vi "Func-엑셀 데이터를 그래프로 출력.vi"() -> ()   [LabVIEW 2015] (continued)
-18.31\t-7.631\n-18.3\t-18.31\t-7.633\n-18.3\t-18.31\t-7.634\n-18.3\t-18.31\t-7.636\n-18.3\t-18.31\t-7.633\n-18.3\t-18.31\t-7.632\n-18.3\t-18.31\t-7.636\n-18.3\t-18.31\t-7.635\n-18.3\t-18.31\t-7.636\n-18.3\t-18.31\t-7.638\n-18.3\t-18.31\t-7.643\n-18.3\t-18.31\t-7.647\n-18.3\t-18.31\t-7.651\n-18.3\t-18.31\t-7.656\n-18.3\t-18.31\t-7.657\n-18.3\t-18.31\t-7.659\n-18.3\t-18.31\t-7.66\n-18.3\t-18.31\t-7.66\n-18.3\t-18.31\t-7.657\n-18.3\t-18.31\t-7.656\n-18.3\t-18.31\t-7.662\n-18.3\t-18.31\t-7.664\n-18.3\t-18.31\t-7.667\n-18.3\t-18.31\t-7.672\n-18.3\t-18.31\t-7.676\n-18.3\t-18.31\t-7.674\n-18.3\t-18.31\t-7.676\n-18.3\t-18.31\t-7.677\n-18.3\t-18.31\t-7.675\n-18.3\t-18.31\t-7.674\n-18.3\t-18.31\t-7.675\n-18.3\t-18.31\t-7.681\n-18.3\t-18.31\t-7.683\n-18.3\t-18.31\t-7.687\n-18.3\t-18.31\t-7.689\n-18.3\t-18.31\t-7.693\n-18.3\t-18.31\t-7.695\n-18.3\t-18.31\t-7.696\n-18.3\t-18.31\t-7.696\n-18.3\t-18.31\t-7.693\n-18.3\t-18.31\t-7.695\n-18.3\t-18.31\t-7.694\n-18.3\t-18.31\t-7.695\n-18.3\t-18.31\t-7.696\n-18.3\t-18.31\t-7.699\n-18.3\t-18.31\t-7.702\n-18.3\t-18.31\t-7.704\n-18.3\t-18.31\t-7.707\n-18.3\t-18.31\t-7.707\n-18.3\t-18.31\t-7.709\n-18.3\t-18.31\t-7.711\n-18.3\t-18.31\t-7.711\n-18.3\t-18.31\t-7.714\n-18.3\t-18.31\t-7.716\n-18.3\t-18.31\t-7.72\n-18.3\t-18.31\t-7.723\n-18.3\t-18.31\t-7.727\n-18.3\t-18.31\t-7.728\n-18.3\t-18.31\t-7.729\n-18.3\t-18.31\t-7.732\n-18.3\t-18.31\t-7.731\n-18.3\t-18.31\t-7.73\n-18.3\t-18.31\t-7.729\n-18.3\t-18.31\t-7.729\n-18.3\t-18.31\t-7.73\n-18.3\t-18.31\t-7.731\n-18.3\t-18.31\t-7.73\n-18.3\t-18.31\t-7.732\n-18.3\t-18.31\t-7.734\n-18.3\t-18.31\t-7.74\n-18.3\t-18.31\t-7.743\n-18.3\t-18.31\t-7.744\n-18.3\t-18.31\t-7.747\n-18.3\t-18.31\t-7.746\n-18.3\t-18.31\t-7.745\n-18.3\t-18.31\t-7.743\n-18.3\t-18.31\t-7.745\n-18.3\t-18.31\t-7.747\n-18.3\t-18.31\t-7.746\n-18.3\t-18.31\t-7.752\n-18.3\t-18.31\t-7.754\n-18.3\t-18.31\t-7.759\n-18.3\t-18.31\t-7.761\n-18.3\t-18.31\t-7.765\n-18.3\t-18.31\t-7.765\n-18.3\t-18.31\t-7.766\n-18.3\t-18.31\t-7.766\n-18.3\t-18.31\t-7.764\n-18.3\t-18.31\t-7.764\n-18.3\t-18.31\t-7.76\n-18.3\t-18.31\t-7.767\n-18.3\t-18.31\t-7.767\n-18.3\t-18.31\t-7.768\n-18.3\t-18.31\t-7.77\n-18.3\t-18.31\t-7.772\n-18.3\t-18.31\t-7.776\n-18.3\t-18.31\t-7.777\n-18.3\t-18.31\t-7.777\n-18.3\t-18.31\t-7.779\n-18.3\t-18.31\t-7.781\n-18.3\t-18.31\t-7.782\n-18.3\t-18.31\t-7.785\n-18.3\t-18.31\t-7.787\n-18.3\t-18.31\t-7.792\n-18.3\t-18.31\t-7.796\n-18.3\t-18.31\t-7.798\n-18.3\t-18.31\t-7.801\n-18.3\t-18.31\t-7.799\n-18.3\t-18.31\t-7.797\n-18.3\t-18.31\t-7.796\n-18.3\t-18.31\t-7.794\n-18.3\t-18.31\t-7.796\n-18.3\t-18.31\t-7.796\n-18.3\t-18.31\t-7.8\n-18.3\t-18.31\t-7.805\n-18.3\t-18.31\t-7.808\n-18.3\t-18.31\t-7.809\n-18.3\t-18.31\t-7.809\n-18.3\t-18.31\t-7.808\n-18.3\t-18.31\t-7.808\n-18.3\t-18.31\t-7.809\n-18.3\t-18.31\t-7.812\n-18.3\t-18.31\t-7.813\n-18.3\t-18.31\t-7.817\n-18.3\t-18.31\t-7.82\n-18.3\t-18.31\t-7.821\n-18.3\t-18.31\t-7.825\n-18.3\t-18.31\t-7.823\n-18.3\t-18.31\t-7.824\n-18.3\t-18.31\t-7.827\n-18.3\t-18.31\t-7.827\n-18.3\t-18.31\t-7.828\n-18.3\t-18.31\t-7.828\n-18.3\t-18.31\t-7.829\n-18.3\t-18.31\t-7.834\n-18.3\t-18.31\t-7.836\n-18.3\t-18.31\t-7.836\n-18.3\t-18.31\t-7.838\n-18.3\t-18.31\t-7.838\n-18.3\t-18.31\t-7.839\n-18.3\t-18.31\t-7.838\n-18.3\t-18.31\t-7.839\n-18.3\t-18.31\t-7.84\n-18.3\t-18.31\t-7.841\n-18.3\t-18.31\t-7.847\n-18.3\t-18.31\t-7.852\n-18.3\t-18.31\t-7.852\n-18.3\t-18.31\t-7.852\n-18.3\t-18.31\t-7.858\n-18.3\t-18.31\t-7.863\n-18.3\t-18.31\t-7.859\n-18.3\t-18.31\t-7.857\n-18.3\t-18.31\t-7.858\n-18.3\t-18.31\t-7.866\n-18.3\t-18.31\t-7.859\n-18.3\t-18.31\t-7.858\n-18.3\t-18.31\t-7.86\n-18.3\t-18.31\t-7.863\n-18.3\t-18.31\t-7.864\n-18.3\t-18.31\t-7.863\n-18.3\t-18.31\t-7.87\n-18.3\t-18.31\t-7.87\n-18.3\t-18.31\t-7.875\n-18.3\t-18.31\t-7.876\n-18.3\t-18.31\t-7.877\n-18.3\t-18.31\t-7.877\n-18.3\t-18.31\t-7.878\n-18.3\t-18.31\t-7.877\n-18.3\t-18.31\t-7.875\n-18.3\t-18.31\t-7.878\n-18.3\t-18.31\t-7.88\n-18.3\t-18.31\t-7.883\n-18.3\t-18.31\t-7.886\n-18.3\t-18.31\t-7.891\n-18.3\t-18.31\t-7.889\n-18.3\t-18.31\t-7.887\n-18.3\t-18.31\t-7.889\n-18.3\t-18.31\t-7.888\n-18.3\t-18.31\t-7.888\n-18.3\t-18.31\t-7.888\n-18.3\t-18.31\t-7.894\n-18.3\t-18.31\t-7.893\n-18.3\t-18.31\t-7.895\n-18.3\t-18.31\t-7.896\n-18.3\t-18.31\t-7.897\n-18.3\t-18.31\t-7.898\n-18.3\t-18.31\t-7.899\n-18.3\t-18.31\t-7.904\n-18.3\t-18.31\t-7.904\n-18.3\t-18.31\t-7.904\n-18.3\t-18.31\t-7.903\n-18.3\t-18.31\t-7.905\n-18.3\t-18.31\t-7.905\n-18.3\t-18.31\t-7.904\n-18.3\t-18.31\t-7.905\n-18.3\t-18.31\t-7.902\n-18.3\t-18.31\t-7.904\n-18.3\t-18.31\t-7.903\n-18.3\t-18.31\t-7.905\n-18.3\t-18.31\t-7.907\n-18.3\t-18.31\t-7.909\n-18.3\t-18.31\t-7.914\n-18.3\t-18.31\t-7.914\n-18.3\t-18.31\t-7.922\n-18.3\t-18.31\t-7.925\n-18.3\t-18.31\t-7.925\n-18.3\t-18.31\t-7.929\n-18.3\t-18.31\t-7.925\n-18.3\t-18.31\t-7.926\n-18.3\t-18.31\t-7.925\n-18.3\t-18.31\t-7.925\n-18.3\t-18.31\t-7.926\n-18.3\t-18.31\t-7.926\n-18.3\t-18.31\t-7.933\n-18.3\t-18.31\t-7.938\n-18.3\t-18.31\t-7.938\n-18.3\t-18.31\t-7.942\n-18.3\t-18.31\t-7.946\n-18.3\t-18.31\t-7.947\n-18.3\t-18.31\t-7.944\n-18.3\t-18.31\t-7.946\n-18.3\t-18.31\t-7.946\n-18.3\t-18.31\t-7.943\n-18.3\t-18.31\t-7.942\n-18.3\t-18.31\t-7.945\n-18.3\t-18.31\t-7.95\n-18.3\t-18.31\t-7.948\n-18.3\t-18.31\t-7.95\n-18.3\t-18.31\t-7.951\n-18.3\t-18.31\t-7.952\n-18.3\t-18.31\t-7.951\n-18.3\t-18.31\t-7.951\n-18.3\t-18.31\t-7.954\n-18.3\t-18.31\t-7.954\n-18.3\t-18.31\t-7.957\n-18.3\t-18.31\t-7.958\n-18.3\t-18.31\t-7.96\n-18.3\t-18.31\t-7.959\n-18.3\t-18.31\t-7.957\n-18.3\t-18.31\t-7.962\n-18.3\t-18.31\t-7.96\n-18.3\t-18.31\t-7.961\n-18.3\t-18.31\t-7.964\n-18.3\t-18.31\t-7.968\n-18.3\t-18.31\t-7.972\n-18.3\t-18.31\t-7.971\n-18.3\t-18.31\t-7.974\n-18.3\t-18.31\t-7.974\n-18.3\t-18.31\t-7.973\n-18.3\t-18.31\t-7.974\n-18.3\t-18.31\t-7.975\n-18.3\t-18.31\t-7.978\n-18.3\t-18.31\t-7.979\n-18.3\t-18.31\t-7.978\n-18.3\t-18.31\t-7.981\n-18.3\t-18.31\t-7.981\n-18.3\t-18.31\t-7.98\n-18.3\t-18.31\t-7.982\n-18.3\t-18.31\t-7.984\n-18.3\t-18.31\t-7.987\n-18.3\t-18.31\t-7.989\n-18.3\t-18.31\t-7.992\n-18.3\t-18.31\t-7.99\n-18.3\t-18.31\t-7.989\n-18.3\t-18.31\t-7.988\n-18.3\t-18.31\t-7.991\n-18.3\t-18.31\t-7.988\n-18.3\t-18.31\t-7.988\n-18.3\t-18.31\t-7.995\n-18.3\t-18.31\t-8\n-18.3\t-18.31\t-7.999\n-18.3\t-18.31\t-7.998\n-18.3\t-18.31\t-8.001\n-18.3\t-18.31\t-8.003\n-18.3\t-18.31\t-8.003\n-18.3\t-18.31\t-8.001\n-18.3\t-18.31\t-8.005\n-18.3\t-18.31\t-8.007\n-18.3\t-18.31\t-8.007\n-18.3\t-18.31\t-8.009\n-18.3\t-18.31\t-8.009\n-18.3\t-18.31\t-8.011\n-18.3\t-18.31\t-8.01\n-18.3\t-18.31\t-8.01\n-18.3\t-18.31\t-8.013\n-18.3\t-18.31\t-8.01\n-18.3\t-18.31\t-8.011\n-18.3\t-18.31\t-8.014\n-18.3\t-18.31\t-8.013\n-18.3\t-18.31\t-8.016\n-18.3\t-18.31\t-8.017\n-18.3\t-18.31\t-8.018\n-18.3\t-18.31\t-8.021\n-18.3\t-18.31\t-8.023\n-18.3\t-18.31\t-8.025\n-18.3\t-18.31\t-8.026\n-18.3\t-18.31\t-8.029\n-18.3\t-18.31\t-8.03\n-18.3\t-18.31\t-8.028\n-18.3\t-18.31\t-8.025\n-18.3\t-18.31\t-8.028\n-18.3\t-18.31\t-8.032\n-18.3\t-18.31\t-8.03\n-18.3\t-18.31\t-8.03\n-18.3\t-18.31\t-8.033\n-18.3\t-18.31\t-8.034\n-18.3\t-18.31\t-8.034\n-18.3\t-18.31\t-8.03\n-18.3\t-18.31\t-8.032\n-18.3\t-18.31\t-8.036\n-18.3\t-18.31\t-8.04\n-18.3\t-18.31\t-8.041\n-18.3\t-18.31\t-8.043\n-18.3\t-18.31\t-8.046\n-18.3\t-18.31\t-8.043\n-18.3\t-18.31\t-8.042\n-18.3\t-18.31\t-8.043\n-18.3\t-18.31\t-8.046\n-18.3\t-18.31\t-8.048\n-18.3\t-18.31\t-8.049\n-18.3\t-18.31\t-8.055\n-18.3\t-18.31\t-8.056\n-18.3\t-18.31\t-8.059\n-18.3\t-18.31\t-8.061\n-18.3\t-18.31\t-8.06\n-18.3\t-18.31\t-8.062\n-18.3\t-18.31\t-8.06\n-18.3\t-18.31\t-8.061\n-18.3\t-18.31\t-8.061\n-18.3\t-18.31\t-8.064\n-18.3\t-18.31\t-8.066\n-18.3\t-18.31\t-8.068\n-18.3\t-18.31\t-8.068\n-18.3\t-18.31\t-8.068\n-18.3\t-18.31\t-8.067\n-18.3\t-18.31\t-8.065\n-18.3\t-18.31\t-8.064\n-18.3\t-18.31\t-8.068\n-18.3\t-18.31\t-8.066\n-18.3\t-18.31\t-8.066\n-18.3\t-18.31\t-8.069\n-18.3\t-18.31\t-8.07\n-18.3\t-18.31\t-8.071\n-18.3\t-18.31\t-8.068\n-18.3\t-18.31\t-8.074\n-18.3\t-18.31\t-8.079\n-18.3\t-18.31\t-8.08\n-18.3\t-18.31\t-8.081\n-18.3\t-18.31\t-8.082\n-18.3\t-18.31\t-8.084\n-18.3\t-18.31\t-8.082\n-18.3\t-18.31\t-8.08\n-18.3\t-18.31\t-8.08\n-18.3\t-18.31\t-8.078\n-18.3\t-18.31\t-8.082\n-18.3\t-18.31\t-8.086\n-18.3\t-18.31\t-8.089\n-18.3\t-18.31\t-8.093\n-18.3\t-18.31\t-8.095\n-18.3\t-18.31\t-8.098\n-18.3\t-18.31\t-8.096\n-18.3\t-18.31\t-8.097\n-18.3\t-18.31\t-8.095\n-18.3\t-18.31\t-8.097\n-18.3\t-18.31\t-8.099\n-18.3\t-18.31\t-8.098\n-18.3\t-18.31\t-8.1\n-18.3\t-18.31\t-8.1\n-18.3\t-18.31\t-8.1\n-18.3\t-18.31\t-8.097\n-18.3\t-18.31\t-8.094\n-18.3\t-18.31\t-8.096\n-18.3\t-18.31\t-8.098\n-18.3\t-18.31\t-8.097\n-18.3\t-18.31\t-8.101\n-18.3\t-18.31\t-8.105\n-18.3\t-18.31\t-8.108\n-18.3\t-18.31\t-8.11\n-18.3\t-18.31\t-8.111\n-18.3\t-18.31\t-8.113\n-18.3\t-18.31\t-8.116\n-18.3\t-18.31\t-8.117\n-18.3\t-18.31\t-8.117\n-18.3\t-18.31\t-8.117\n-18.3\t-18.31\t-8.116\n-18.3\t-18.31\t-8.118\n-18.3\t-18.31\t-8.12\n-18.3\t-18.31\t-8.125\n-18.3\t-18.31\t-8.125\n-18.3\t-18.31\t-8.127\n-18.3\t-18.31\t-8.132\n-18.3\t-18.31\t-8.131\n-18.3\t-18.31\t-8.13\n-18.3\t-18.31\t-8.128\n-18.3\t-18.31\t-8.129\n-18.3\t-18.31\t-8.125\n-18.3\t-18.31\t-8.125\n-18.3\t-18.31\t-8.125\n-18.3\t-18.31\t-8.124\n-18.3\t-18.31\t-8.126\n-18.3\t-18.31\t-8.126\n-18.3\t-18.31\t-8.132\n-18.3\t-18.31\t-8.134\n-18.3\t-18.31\t-8.136\n-18.3\t-18.31\t-8.136\n-18.3\t-18.31\t-8.134\n-18.3\t-18.31\t-8.136\n-18.3\t-18.31\t-8.132\n-18.3\t-18.31\t-8.13\n-18.3\t-18.31\t-8.131\n-18.3\t-18.31\t-8.135\n-18.3\t-18.31\t-8.139\n-18.3\t-18.31\t-8.138\n-18.3\t-18.31\t-8.14\n-18.3\t-18.31\t-8.143\n-18.3\t-18.31\t-8.144\n-18.3\t-18.31\t-8.144\n-18.3\t-18.31\t-8.145\n-18.3\t-18.31\t-8.145\n-18.3\t-18.31\t-8.149\n-18.3\t-18.31\t-8.15\n-18.3\t-18.31\t-8.148\n-18.3\t-18.31\t-8.148\n-18.3\t-18.31\t-8.145\n-18.3\t-18.31\t-8.147\n-18.3\t-18.31\t-8.146\n-18.3\t-18.31\t-8.15\n-18.3\t-18.31\t-8.154\n-18.3\t-18.31\t-8.154\n-18.3\t-18.31\t-8.16\n-18.3\t-18.31\t-8.16\n-18.3\t-18.31\t-8.159\n-18.3\t-18.31\t-8.158\n-18.3\t-18.31\t-8.154\n-18.3\t-18.31\t-8.155\n-18.3\t-18.31\t-8.155\n-18.3\t-18.31\t-8.157\n-18.3\t-18.31\t-8.159\n-18.3\t-18.31\t-8.159\n-18.3\t-18.31\t-8.161\n-18.3\t-18.31\t-8.163\n-18.3\t-18.31\t-8.162\n-18.3\t-18.31\t-8.163\n-18.3\t-18.31\t-8.164\n-18.3\t-18.31\t-8.164\n-18.3\t-18.31\t-8.168\n-18.3\t-18.31\t-8.166\n-18.3\t-18.31\t-8.168\n-18.3\t-18.31\t-8.17\n-18.3\t-18.31\t-8.174\n-18.3\t-18.31\t-8.174\n-18.3\t-18.31\t-8.174\n-18.3\t-18.31\t-8.177\n-18.3\t-18.31\t-8.18\n-18.3\t-18.31\t-8.181\n-18.3\t-18.31\t-8.179\n-18.3\t-18.31\t-8.178\n-18.3\t-18.31\t-8.177\n-18.3\t-18.31\t-8.178\n-18.3\t-18.31\t-8.177\n-18.3\t-18.31\t-8.175\n-18.3\t-18.31\t-8.178\n-18.3\t-18.31\t-8.181\n-18.3\t-18.31\t-8.186\n-18.3\t-18.31\t-8.185\n-18.3\t-18.31\t-8.188\n-18.3\t-18.31\t-8.189\n-18.3\t-18.31\t-8.189\n-18.3\t-18.31\t-8.186\n-18.3\t-18.31\t-8.184\n-18.3\t-18.31\t-8.187\n-18.3\t-18.31\t-8.187\n-18.3\t-18.31\t-8.189\n-18.3\t-18.31\t-8.19\n-18.3\t-18.31\t-8.195\n-18.3\t-18.31\t-8.197\n-18.3\t-18.31\t-8.197\n-18.3\t-18.31\t-8.196\n-18.3\t-18.31\t-8.197\n-18.3\t-18.31\t-8.198\n-18.3\t-18.31\t-8.201\n-18.3\t-18.31\t-8.202\n-18.3\t-18.31\t-8.205\n-18.3\t-18.31\t-8.207\n-18.3\t-18.31\t-8.209\n-18.3\t-18.31\t-8.211\n-18.3\t-18.31\t-8.209\n-18.3\t-18.31\t-8.211\n-18.3\t-18.31\t-8.209\n-18.3\t-18.31\t-8.207\n-18.3\t-18.31\t-8.21\n-18.3\t-18.31\t-8.212\n-18.3\t-18.31\t-8.216\n-18.3\t-18.31\t-8.216\n-18.3\t-18.31\t-8.215\n-18.3\t-18.31\t-8.22\n-18.3\t-18.31\t-8.218\n-18.3\t-18.31\t-8.214\n-18.3\t-18.31\t-8.214\n-18.3\t-18.31\t-8.213\n-18.3\t-18.31\t-8.214\n-18.3\t-18.31\t-8.213\n-18.3\t-18.31\t-8.213\n-18.3\t-18.31\t-8.218\n-18.3\t-18.31\t-8.218\n-18.3\t-18.31\t-8.22\n-18.3\t-18.31\t-8.226\n-18.3\t-18.31\t-8.226\n-18.3\t-18.31\t-8.229\n-18.3\t-18.31\t-8.229\n-18.3\t-18.31\t-8.229\n-18.3\t-18.31\t-8.229\n-18.3\t-18.31\t-8.226\n-18.3\t-18.31\t-8.226\n-18.3\t-18.31\t-8.224\n-18.3\t-18.31\t-8.221\n-18.3\t-18.31\t-8.225\n-18.3\t-18.31\t-8.225\n-18.3\t-18.31\t-8.233\n-18.3\t-18.31\t-8.232\n-18.3\t-18.31\t-8.234\n-18.3\t-18.31\t-8.238\n-18.3\t-18.31\t-8.235\n-18.3\t-18.31\t-8.236\n-18.3\t-18.31\t-8.23\n-18.3\t-18.31\t-8.234\n-18.3\t-18.31\t-8.234\n-18.3\t-18.31\t-8.233\n-18.3\t-18.31\t-8.237\n-18.3\t-18.31\t-8.239\n-18.3\t-18.31\t-8.241\n-18.3\t-18.31\t-8.24\n-18.3\t-18.31\t-8.24\n-18.3\t-18.31\t-8.241\n-18.3\t-18.31\t-8.241\n-18.3\t-18.31\t-8.243\n-18.3\t-18.31\t-8.244\n-18.3\t-18.31\t-8.245\n-18.3\t-18.31\t-8.249\n-18.3\t-18.31\t-8.251\n-18.3\t-18.31\t-8.248\n-18.3\t-18.31\t-8.245\n-18.3\t-18.31\t-8.249\n-18.3\t-18.31\t-8.252\n-18.3\t-18.31\t-8.25\n-18.3\t-18.31\t-8.251\n-18.3\t-18.31\t-8.253\n-18.3\t-18.31\t-8.255\n-18.3\t-18.31\t-8.254\n-18.3\t-18.31\t-8.254\n-18.3\t-18.31\t-8.254\n-18.3\t-18.31\t-8.257\n-18.3\t-18.31\t-8.258\n-18.3\t-18.31\t-8.257\n-18.3\t-18.31\t-8.259\n-18.3\t-18.31\t-8.262\n-18.3\t-18.31\t-8.265\n-18.3\t-18.31\t-8.263\n-18.3\t-18.31\t-8.265\n-18.3\t-18.31\t-8.268\n-18.3\t-18.31\t-8.272\n-18.3\t-18.31\t-8.272\n-18.3\t-18.31\t-8.272\n-18.3\t-18.31\t-8.272\n-18.3\t-18.31\t-8.271\n-18.3\t-18.31\t-8.268\n-18.3\t-18.31\t-8.266\n-18.3\t-18.31\t-8.268\n-18.3\t-18.31\t-8.27\n-18.3\t-18.31\t-8.273\n-18.3\t-18.31\t-8.273\n-18.3\t-18.31\t-8.275\n-18.3\t-18.31\t-8.273\n-18.3\t-18.31\t-8.271\n-18.3\t-18.31\t-8.273\n-18.3\t-18.31\t-8.277\n-18.3\t-18.31\t-8.279\n-18.3\t-18.31\t-8.28\n-18.3\t-18.31\t-8.287\n-18.3\t-18.31\t-8.285\n-18.3\t-18.31\t-8.284\n-18.3\t-18.31\t-8.281\n-18.3\t-18.31\t-8.283\n-18.3\t-18.31\t-8.281\n-18.3\t-18.31\t-8.279\n-18.3\t-18.31\t-8.282\n-18.3\t-18.31\t-8.284\n-18.3\t-18.31\t-8.287\n-18.3\t-18.31\t-8.288\n-18.3\t-18.31\t-8.288\n-18.3\t-18.31\t-8.291\n-18.3\t-18.31\t-8.293\n-18.3\t-18.31\t-8.293\n-18.3\t-18.31\t-8.291\n-18.3\t-18.31\t-8.29\n-18.3\t-18.31\t-8.291\n-18.3\t-18.31\t-8.288\n-18.3\t-18.31\t-8.284\n-18.3\t-18.31\t-8.285\n-18.3\t-18.31\t-8.29\n-18.3\t-18.31\t-8.289\n-18.3\t-18.31\t-8.29\n-18.3\t-18.31\t-8.292\n-18.3\t-18.31\t-8.294\n-18.3\t-18.31\t-8.295\n-18.3\t-18.31\t-8.292\n-18.3\t-18.31\t-8.295\n-18.3\t-18.31\t-8.297\n-18.3\t-18.31\t-8.296\n-18.3\t-18.31\t-8.297\n-18.3\t-18.31\t-8.3\n-18.3\t-18.31\t-8.303\n-18.3\t-18.31\t-8.304\n-18.3\t-18.31\t-8.304\n-18.3\t-18.31\t-8.309\n-18.3\t-18.31\t-8.312\n-18.3\t-18.31\t-8.313\n-18.3\t-18.31\t-8.31\n-18.3\t-18.31\t-8.31\n-18.3\t-18.31\t-8.312\n-18.3\t-18.31\t-8.309\n-18.3\t-18.31\t-8.307\n-18.3\t-18.31\t-8.309\n-18.3\t-18.31\t-8.313\n-18.3\t-18.31\t-8.314\n-18.3\t-18.31\t-8.316\n-18.3\t-18.31\t-8.321\n-18.3\t-18.31\t-8.322\n-18.3\t-18.31\t-8.32\n-18.3\t-18.31\t-8.32\n-18.3\t-18.31\t-8.32\n-18.3\t-18.31\t-8.32\n-18.3\t-18.31\t-8.318\n-18.3\t-18.31\t-8.32\n-18.3\t-18.31\t-8.32\n-18.3\t-18.31\t-8.322\n-18.3\t-18.31\t-8.323\n-18.3\t-18.31\t-8.323\n-18.3\t-18.31\t-8.323\n-18.3\t-18.31\t-8.324\n-18.3\t-18.31\t-8.324\n-18.3\t-18.31\t-8.321\n-18.3\t-18.31\t-8.319\n-18.3\t-18.31\t-8.32\n-18.3\t-18.31\t-8.319\n-18.3\t-18.31\t-8.316\n-18.3\t-18.31\t-8.318\n-18.3\t-18.31\t-8.32\n-18.3\t-18.31\t-8.321\n-18.3\t-18.31\t-8.323\n-18.3\t-18.31\t-8.326\n-18.3\t-18.31\t-8.33\n-18.3\t-18.31\t-8.334\n-18.3\t-18.31\t-8.336\n-18.3\t-18.31\t-8.337\n-18.3\t-18.31\t-8.341\n-18.3\t-18.31\t-8.339\n-18.3\t-18.31\t-8.341\n-18.3\t-18.31\t-8.34\n-18.3\t-18.31\t-8.34\n-18.3\t-18.31\t-8.342\n-18.3\t-18.31\t-8.339\n-18.3\t-18.31\t-8.341\n-18.3\t-18.31\t-8.339\n-18.3\t-18.31\t-8.341\n-18.3\t-18.31\t-8.34\n-18.3\t-18.31\t-8.343\n-18.3\t-18.31\t-8.341\n-18.3\t-18.31\t-8.339\n-18.3\t-18.31\t-8.34\n-18.3\t-18.31\t-8.341\n-18.3\t-18.31\t-8.342\n-18.3\t-18.31\t-8.339\n-18.3\t-18.31\t-8.346\n-18.3\t-18.31\t-8.348\n-18.3\t-18.31\t-8.348\n-18.3\t-18.31\t-8.349\n-18.3\t-18.31\t-8.354\n-18.3\t-18.31\t-8.354\n-18.3\t-18.31\t-8.352\n-18.3\t-18.31\t-8.355\n-18.3\t-18.31\t-8.357\n-18.3\t-18.31\t-8.358\n-18.3\t-18.31\t-8.354\n-18.3\t-18.31\t-8.357\n-18.3\t-18.31\t-8.358\n-18.3\t-18.31\t-8.356\n-18.3\t-18.31\t-8.354\n-18.3\t-18.31\t-8.354\n-18.3\t-18.31\t-8.355\n-18.3\t-18.31\t-8.357\n-18.3\t-18.31\t-8.357\n-18.3\t-18.31\t-8.361\n-18.3\t-18.31\t-8.364\n-18.3\t-18.31\t-8.365\n-18.3\t-18.31\t-8.366\n-18.3\t-18.31\t-8.366\n-18.3\t-18.31\t-8.368\n-18.3\t-18.31\t-8.366\n-18.3\t-18.31\t-8.367\n-18.3\t-18.31\t-8.363\n-18.3\t-18.31\t-8.365\n-18.3\t-18.31\t-8.364\n-18.3\t-18.31\t-8.363\n-18.3\t-18.31\t-8.364\n-18.3\t-18.31\t-8.366\n-18.3\t-18.31\t-8.366\n-18.3\t-18.31\t-8.367\n-18.3\t-18.31\t-8.368\n-18.3\t-18.31\t-8.369\n-18.3\t-18.31\t-8.369\n-18.3\t-18.31\t-8.373\n-18.3\t-18.31\t-8.376\n-18.3\t-18.31\t-8.376\n-18.3\t-18.31\t-8.377\n-18.3\t-18.31\t-8.382\n-18.3\t-18.31\t-8.385\n-18.3\t-18.31\t-8.384\n-18.3\t-18.31\t-8.387\n-18.3\t-18.31\t-8.388\n-18.3\t-18.31\t-8.389\n-18.3\t-18.31\t-8.388\n-18.3\t-18.31\t-8.384\n-18.3\t-18.31\t-8.38\n-18.3\t-18.31\t-8.377\n-18.3\t-18.31\t-8.377\n-18.3\t-18.31\t-8.378\n-18.3\t-18.31\t-8.377\n-18.3\t-18.31\t-8.379\n-18.3\t-18.31\t-8.381\n-18.3\t-18.31\t-8.382\n-18.3\t-18.31\t-8.384\n-18.3\t-18.31\t-8.386\n-18.3\t-18.31\t-8.389\n-18.3\t-18.31\t-8.388\n-18.3\t-18.31\t-8.389\n-18.3\t-18.31\t-8.39\n-18.3\t-18.31\t-8.391\n-18.3\t-18.31\t-8.387\n-18.3\t-18.31\t-8.388\n-18.3\t-18.31\t-8.39\n-18.3\t-18.31\t-8.391\n-18.3\t-18.31\t-8.391\n-18.3\t-18.31\t-8.388\n-18.3\t-18.31\t-8.391\n-18.3\t-18.31\t-8.391\n-18.3\t-18.31\t-8.39\n-18.3\t-18.31\t-8.387\n-18.3\t-18.31\t-8.39\n-18.3\t-18.31\t-8.393\n-18.3\t-18.31\t-8.395\n-18.3\t-18.31\t-8.392\n-18.3\t-18.31\t-8.395\n-18.3\t-18.31\t-8.402\n-18.3\t-18.31\t-8.4\n-18.3\t-18.31\t-8.399\n-18.3\t-18.31\t-8.4\n-18.3\t-18.31\t-8.402\n-18.3\t-18.31\t-8.4\n-18.3\t-18.31\t-8.401\n-18.3\t-18.31\t-8.403\n-18.3\t-18.31\t-8.406\n-18.3\t-18.31\t-8.4\n-18.3\t-18.31\t-8.405\n-18.3\t-18.31\t-8.408\n-18.3\t-18.31\t-8.405\n-18.3\t-18.31\t-8.406\n-18.3\t-18.31\t-8.404\n-18.3\t-18.31\t-8.406\n-18.3\t-18.31\t-8.404\n-18.3\t-18.31\t-8.404\n-18.3\t-18.31\t-8.405\n-18.3\t-18.31\t-8.405\n-18.3\t-18.31\t-8.408\n-18.3\t-18.31\t-8.409\n-18.3\t-18.31\t-8.411\n-18.3\t-18.31\t-8.412\n-18.3\t-18.31\t-8.414\n-18.3\t-18.31\t-8.413\n-18.3\t-18.31\t-8.413\n-18.3\t-18.31\t-8.416\n-18.3\t-18.31\t-8.419\n-18.3\t-18.31\t-8.419\n-18.3\t-18.31\t-8.418\n-18.3\t-18.31\t-8.418\n-18.3\t-18.31\t-8.415\n-18.3\t-18.31\t-8.413\n-18.3\t-18.31\t-8.41\n-18.3\t-18.31\t-8.408\n-18.3\t-18.31\t-8.41\n-18.3\t-18.31\t-8.414\n-18.3\t-18.31\t-8.418\n-18.3\t-18.31\t-8.42\n-18.3\t-18.31\t-8.418\n-18.3\t-18.31\t-8.42\n-18.3\t-18.31\t-8.42\n-18.3\t-18.31\t-8.42\n-18.3\t-18.31\t-8.42\n-18.3\t-18.31\t-8.42\n-18.3\t-18.31\t-8.425\n-18.3\t-18.31\t-8.43\n-18.3\t-18.31\t-8.427\n-18.3\t-18.31\t-8.429\n-18.3\t-18.31\t-8.429\n-18.3\t-18.31\t-8.428\n-18.3\t-18.31\t-8.428\n-18.3\t-18.31\t-8.426\n-18.3\t-18.31\t-8.428\n-18.3\t-18.31\t-8.425\n-18.3\t-18.31\t-8.424\n-18.3\t-18.31\t-8.426\n-18.3\t-18.31\t-8.429\n-18.3\t-18.31\t-8.43\n-18.3\t-18.31\t-8.432\n-18.3\t-18.31\t-8.435\n-18.3\t-18.31\t-8.436\n-18.3\t-18.31\t-8.435\n-18.3\t-18.31\t-8.433\n-18.3\t-18.31\t-8.43\n-18.3\t-18.31\t-8.427\n-18.3\t-18.31\t-8.429\n-18.3\t-18.31\t-8.434\n-18.3\t-18.31\t-8.436\n-18.3\t-18.31\t-8.439\n-18.3\t-18.31\t-8.442\n-18.3\t-18.31\t-8.444\n-18.3\t-18.31\t-8.45\n-18.3\t-18.31\t-8.448\n-18.3\t-18.31\t-8.447\n-18.3\t-18.31\t-8.445\n-18.3\t-18.31\t-8.445\n-18.3\t-18.31\t-8.443\n-18.3\t-18.31\t-8.437\n-18.3\t-18.31\t-8.437\n-18.3\t-18.31\t-8.441\n-18.3\t-18.31\t-8.443\n-18.3\t-18.31\t-8.441\n-18.3\t-18.31\t-8.44\n-18.3\t-18.31\t-8.445\n-18.3\t-18.31\t-8.448\n-18.3\t-18.31\t-8.443\n-18.3\t-18.31\t-8.442\n-18.3\t-18.31\t-8.446\n-18.3\t-18.31\t-8.452\n-18.3\t-18.31\t-8.45\n-18.3\t-18.31\t-8.446\n-18.3\t-18.31\t-8.447\n-18.3\t-18.31\t-8.45\n-18.3\t-18.31\t-8.448\n-18.3\t-18.31\t-8.448\n-18.3\t-18.31\t-8.449\n-18.3\t-18.31\t-8.453\n-18.3\t-18.31\t-8.454\n-18.3\t-18.31\t-8.454\n-18.3\t-18.31\t-8.458\n-18.3\t-18.31\t-8.461\n-18.3\t-18.31\t-8.464\n-18.3\t-18.31\t-8.466\n-18.3\t-18.31\t-8.468\n-18.3\t-18.31\t-8.473\n-18.3\t-18.31\t-8.471\n-18.3\t-18.31\t-8.471\n-18.3\t-18.31\t-8.469\n-18.3\t-18.31\t-8.467\n-18.3\t-18.31\t-8.465\n-18.3\t-18.31\t-8.461\n-18.3\t-18.31\t-8.457\n-18.3\t-18.31\t-8.455\n-18.3\t-18.31\t-8.455\n-18.3\t-18.31\t-8.457\n-18.3\t-18.31\t-8.46\n-18.3\t-18.31\t-8.461\n-18.3\t-18.31\t-8.466\n-18.3\t-18.31\t-8.47\n-18.3\t-18.31\t-8.47\n
